vi "userauth_publickey_frommemory.vi"() -> ()   [LabVIEW 2017]
doc: "Illustrates how to authenticate a session using public key, read from memory."
uses:
  libssh2/libssh2_session_handshake_tcp.vi
  libssh2/libssh2_init_default.vi
  libssh2/libssh2_session_init_ex.vi
  <vilib>/Utility/tcp.llb/TCP Get Raw Net Object.vi
  libssh2/libssh2_session_handshake_socket.vi
  libssh2/libssh2.lvlib
panel:
  out "authenticated":bool
  in  "private key data":string
  in  "public key data":string
  in  "passphrase":string
  in  "username":string
  in  "hostname":string="localhost"
  out "error out":errorcluster
  # "This is the public key (e.g., generated with ssh-keygen)"
  # "This is the private key (e.g., generated with ssh-keygen)\n\nImportant: If your keys don't work, try generating keys\nwith the following command: \"ssh-keygen -m PEM -t rsa\".\nThis will create a key with the header\n\"-----BEGIN RSA PRIVATE KEY-----\" as is expected by libssh2."
  # "This is the passphrase for your private key."
  # "When everything goes right, this status should be TRUE."
  # "Important\nThis only works when libssh2 is backed by OpenSSL. You can verify the crypo-library of your version\nof libssh2 with libssh2_crypto_engine.vi"
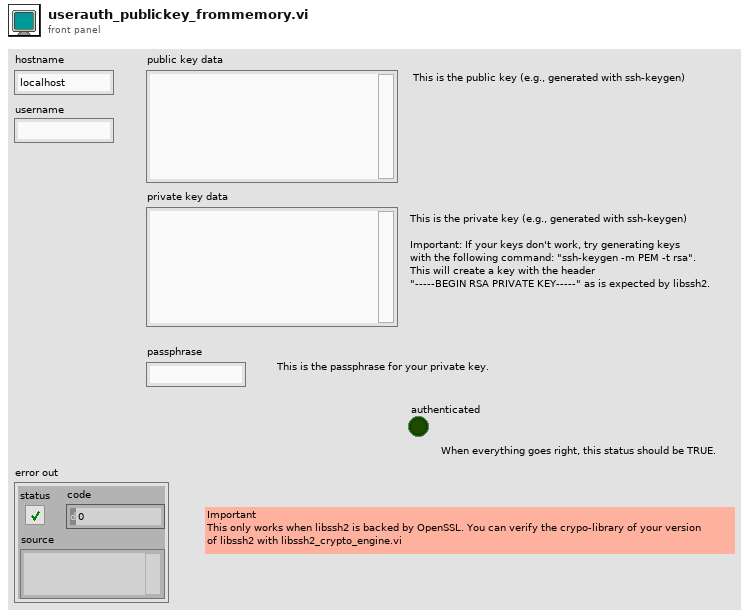
[diagram p1: front panel]
types:
  T1 = typedef "libssh2.lvlib/Session Refnum.ctl" = refnum<k1>
  T2 = typedef "libssh2.lvlib/libssh2_crypto_engine.ctl" = enum16{"no crypto", "OpenSSL", "gcrypt", "mbedTLS", "WinCNG", "OS400qc3"}
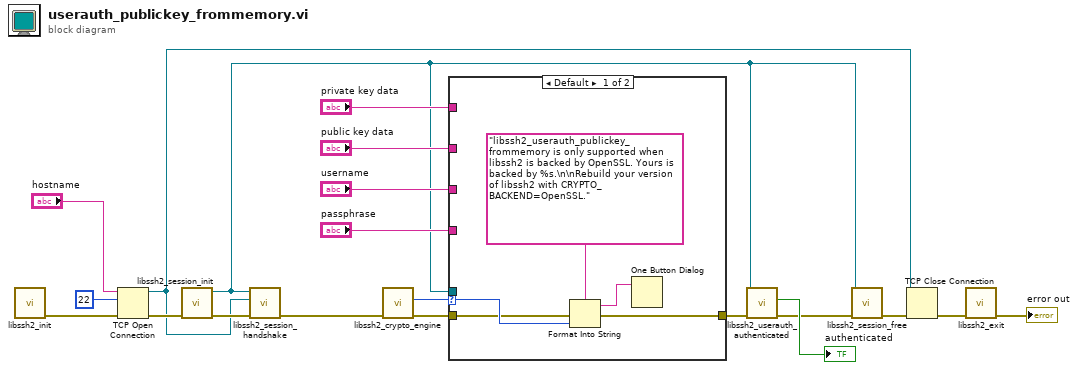
[diagram p0: block diagram]
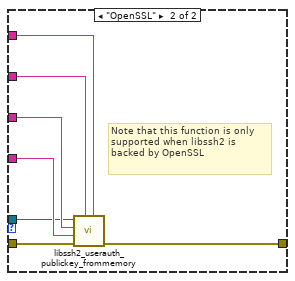
[diagram p2: hidden frame]
diagram:
  n1 = call-poly "libssh2_init.vi"() -> ("error out"=w20:errorcluster)  [unwired: 11 in]
  n2 = TCP Open Connection(address="hostname", remote port or service name=u16 22, error in (no error)=w20) -> (connection ID=w11:refnum<k5>, error out=w12:errorcluster)  [unwired: 2 in]
  n3 = call "libssh2_session_init.vi"("error in (no error)"=w12) -> ("error out"=w15:errorcluster, "session"=w2:T1)  [unwired: 9 in]
  n4 = call-poly "libssh2_session_handshake.vi"("error in (no error)"=w15, "tcp connection"=w11, "session"=w2) -> ("error out"=w4:errorcluster)  [unwired: 8 in]
  n5 = call "libssh2_crypto_engine.vi"("error in (no error)"=w4) -> ("error out"=w3:errorcluster, "crypto engine"=w1:T2)  [unwired: 9 in]
  n6 = case shown="Default" w1 {
    selector: w1 -> [w24 _]
    tunnel: "username" -> [_ w32]
    tunnel: [w22 w31] -> w10
    tunnel: "passphrase" -> [_ w30]
    tunnel: "public key data" -> [_ w29]
    tunnel: "private key data" -> [_ w28]
    tunnel: w3 -> [w23 w27]
    tunnel: w2 -> [_ w26]
    frame Default {
      n7 = Format Into String(format string="libssh2_userauth_publickey_frommemory is only supported when libssh2 is backed by OpenSSL. Yours is backed by %s.\n\nRebuild your version of libssh2 with CRYPTO_BACKEND=OpenSSL.", error in=w23, w24) -> (resulting string=w21:string, error out=w22:errorcluster)  [unwired: 1 in]
      n8 = One Button Dialog(message=w21) -> ()  [unwired: 1 in, 1 out]
    }
    frame "OpenSSL" {
      # "Note that this function is only supported when libssh2 is backed by OpenSSL"
      n9 = call "libssh2_userauth_publickey_frommemory.vi"("private key data"=w28, "public key data"=w29, "error in (no error)"=w27, "passphrase"=w30, "username"=w32, "session"=w26) -> ("error out"=w31:errorcluster)  [unwired: 5 in]
    }
  }
  n10 = call "libssh2_userauth_authenticated.vi"("error in (no error)"=w10, "session"=w2) -> ("error out"=w7:errorcluster, "authenticated"=→"authenticated":bool)  [unwired: 8 in]
  n11 = call "libssh2_session_free.vi"("error in (no error)"=w7, "session"=w2) -> ("error out"=w13:errorcluster)  [unwired: 9 in]
  n12 = TCP Close Connection(connection ID=w11, error in (no error)=w13) -> (error out=w17:errorcluster)  [unwired: 1 in, 1 out]
  n13 = call "libssh2_exit.vi"("error in (no error)"=w17) -> ("error out"=→"error out":errorcluster)  [unwired: 10 in]
